vi "action.vi"(0 "HGF_TaskEventListener":refnum<class "HGF_TaskEventListener.lvclass">, 5 "error in (no error)":errorcluster, 8 "HGF_ThreadWorker":refnum<class "HGF_ThreadWorker.lvclass">) -> (10 "dup HGF_ThreadWorker":refnum<class "HGF_ThreadWorker.lvclass">, 14 "dup HGF_TaskEventListener":refnum<class "HGF_TaskEventListener.lvclass">, 19 "error out":errorcluster)   [LabVIEW 2012, in "HGF_ObjectManager.lvlib" / "HGF_TaskEventListener.lvclass"]
doc: "This is a dynamic dispatch VI that is called from Visitor.visit(). It will call member VIs of Visitable to perform the requested action which means: calling public methods of Visitable child class.\n\n<B>Hint:</B> This method is abstract and need to be implemented by child classes."
uses:
  HGF_TaskEventListener.lvclass
  HGF_ThreadWorker/HGF_ThreadWorker.lvclass
  HGF_Stop/HGF_Stop.lvclass
  HGF_NetworkVisitor/HGF_NetworkVisitor.lvclass
  HGF_Event/HGF_Event.lvclass
  HGF_Visitable/HGF_Visitable.lvclass
  HGF_ThreadTask/HGF_ThreadTask.lvclass
  HGF_Visitor/HGF_Visitor.lvclass
  HGF_ObjectManager/HGF_ObjectManager.lvlib
  HGF_Reference/HGF_Reference.lvclass
  HGF_Exception/HGF_Exception.lvclass
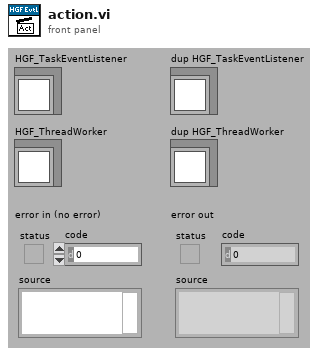
[diagram p1: front panel]
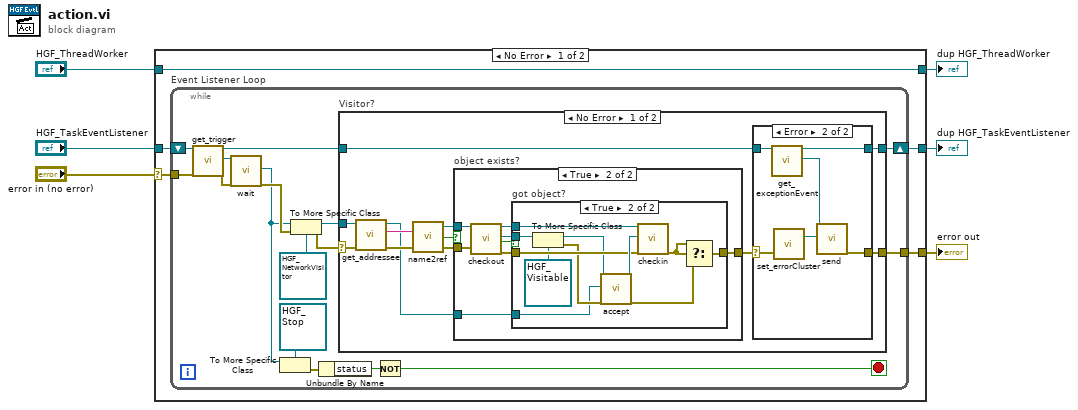
[diagram p0: block diagram]
diagram:
  n1 = case shown="No Error" "error in (no error)" {
    selector: "error in (no error)" -> [w7 w72]
    tunnel: "HGF_TaskEventListener" -> [w8 w73]
    tunnel: [w11 w73] -> w2
    tunnel: [w10 w72] -> w1
    tunnel: [w9 w71] -> w3
    tunnel: "HGF_ThreadWorker" -> [w9 w71]
    frame No Error {
      n2 = while "Event Listener Loop" {
        tunnel: [w18] -> w10
        shift-right: [w27] -> w11
        shift-left: w8 -> [w25]
        tunnel: w7 -> [w23]
        stop <- w13 stop-if-true
        n3 = call "get_trigger.vi"("HGF_ThreadTask"=w25, "error in (no error)"=w23) -> ("dup HGF_ThreadTask"=w24:refnum<class "HGF_TaskEventListener.lvclass">, "trigger"=w21:refnum<class "HGF_Event.lvclass">, "error out"=w22:errorcluster)  [unwired: 15 out]
        n4 = call-dynamic "wait.vi"("HGF_Event"=w21, "error in (no error)"=w22) -> ("Object"=w16:refnum<class>, "error out"=w26:errorcluster)  [unwired: 2 in, 14 out]
        n5 = To More Specific Class(target class=refnum<class "HGF_Stop.lvclass"> refnum ("HGF_BaseClasses.lvlib:HGF_Stop.lvclass"), reference=w16) -> (error out=w15:errorcluster)  [unwired: 1 in, 1 out]
        n6 = To More Specific Class(target class=refnum<class "HGF_NetworkVisitor.lvclass"> refnum ("HGF_BaseClasses.lvlib:HGF_NetworkData.lvclass"), reference=w16, error in=w26) -> (specific class reference=w20:refnum<class "HGF_NetworkVisitor.lvclass">, error out=w19:errorcluster)
        n7 = Unbundle By Name(w15) -> ("status"=w14:bool)
        n8 = case "Visitor?" shown="No Error" w19 {
          selector: w19 -> [w36 w69]
          tunnel: [w38 w69] -> w18
          tunnel: w24 -> [w33 w70]
          tunnel: [w39 w70] -> w27
          tunnel: w20 -> [w37 _]
          frame No Error {
            n9 = call "get_addressee.vi"("error in (no error)"=w36, "HGF_Visitor"=w37) -> ("error out"=w35:errorcluster, "addressee"=w34:string, "dup HGF_Visitor"=w29:refnum<class "HGF_NetworkVisitor.lvclass">)  [unwired: 7 out]
            n10 = call "name2ref.vi"("error in (no error)"=w35, "name"=w34) -> ("error out"=w31:errorcluster, "obj exists"=w30:bool, "objectRef out"=w32:refnum<class "HGF_Reference.lvclass">)  [unwired: 1 out]
            n11 = case "object exists?" shown="True" w30 {
              tunnel: w32 -> [_ w48]
              tunnel: w31 -> [w40 w47]
              tunnel: w29 -> [_ w42]
              tunnel: [w40 w41] -> w28
              frame False {
              }
              frame True {
                n12 = call "checkout.vi"("HGF_Reference"=w48, "error in (no error)"=w47) -> ("dup HGF_Reference"=w44:refnum<class "HGF_Reference.lvclass">, "Object"=w43:refnum<class>, "got object?"=w46:bool, "error out"=w45:errorcluster)  [unwired: 1 in, 13 out]
                n13 = case "got object?" shown="True" w46 {
                  tunnel: w45 -> [w49 w57]
                  tunnel: w44 -> [_ w60]
                  tunnel: w43 -> [_ w58]
                  tunnel: w42 -> [_ w53]
                  tunnel: [w49 w50] -> w41
                  frame False {
                  }
                  frame True {
                    n14 = To More Specific Class(target class=refnum<class "HGF_Visitable.lvclass"> refnum ("HGF_BaseClasses.lvlib:HGF_Visitable.lvclass"), reference=w58) -> (specific class reference=w55:refnum<class "HGF_Visitable.lvclass">, error out=w54:errorcluster)  [unwired: 1 in]
                    n15 = call "accept.vi"("HGF_Visitable"=w55, "HGF_Visitor"=w53, "error in (no error)"=w54) -> ("dup HGF_Visitable"=w59:refnum<class "HGF_Visitable.lvclass">, "error out"=w51:errorcluster)  [unwired: 15 out]
                    n16 = call "checkin.vi"("HGF_Reference"=w60, "Object"=w59, "error in (no error)"=w57) -> ("error out"=w52:errorcluster)  [unwired: 1 in, 15 out]
                    n17 = Select(t=w52, s=w52, f=w51) -> (s? t:f=w50:errorcluster)
                  }
                }
              }
            }
            n18 = case shown="Error" w28 {
              selector: w28 -> [w61 w67]
              tunnel: [w62 w64] -> w39
              tunnel: [w61 w68] -> w38
              tunnel: w33 -> [w62 w65]
              frame No Error {
              }
              frame Error {
                n19 = call "get_exceptionEvent.vi"("HGF_ThreadTask"=w65) -> ("dup HGF_ThreadTask"=w64:refnum<class "HGF_TaskEventListener.lvclass">, "exceptionEvent"=w63:refnum<class "HGF_Event.lvclass">)  [unwired: 1 in, 16 out]
                n20 = call "set_errorCluster.vi"("error in (no error)"=w67) -> ("dup HGF_Exception"=w66:refnum<class "HGF_Exception.lvclass">)  [unwired: 1 in]
                n21 = call-dynamic "send.vi"("HGF_Event"=w63, "Object"=w66) -> ("error out"=w68:errorcluster)  [unwired: 3 in, 14 out]
              }
            }
          }
          frame Error {
          }
        }
        n22 = Not(x=w14) -> (.not. x?=w13:bool)
      }
    }
    frame Error {
    }
  }
  "error out" <- w1
  "dup HGF_TaskEventListener" <- w2
  "dup HGF_ThreadWorker" <- w3
